vi "Compare.vi"(4 "gB":dbl, 6 "fB":dbl, 9 "gA":dbl, 10 "fA":dbl, 11 "Priority Queue in":refnum<class "NI_Robotics_Priority Queue.lvclass">) -> (2 "priority(A) > priority(B)":bool, 3 "Priority Queue out":refnum<class "NI_Robotics_Priority Queue.lvclass">)   [LabVIEW 2017, in "NI_Robotics_Priority Queue.lvclass"]
uses:
  <vilib>/robotics/Navigation/shared/Priority Queue/NI_Robotics_Priority Queue.lvclass
  <vilib>/robotics/Navigation/shared/Priority Queue/NI_Robotics_Priority Queue.lvclass/NI_Robotics_Priority Queue.ctl
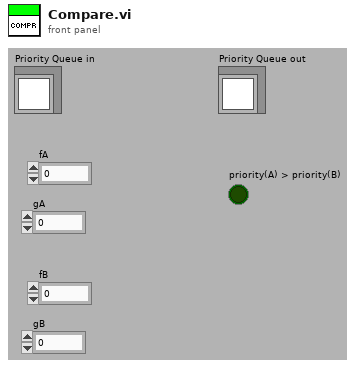
[diagram p1: front panel]
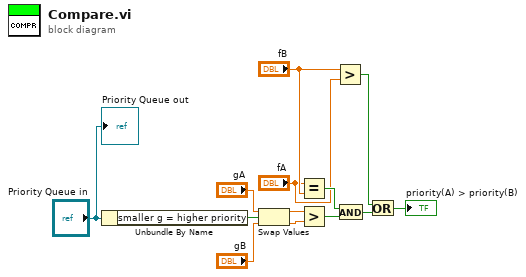
[diagram p0: block diagram]
diagram:
  n1 = Unbundle By Name("Priority Queue in") -> ("smaller g = higher priority"=w13:bool)
  n2 = Swap Values(12:"gA", 13:w13, 14:"gB") -> (1:w5:dbl, 3:w4:dbl)
  n3 = Equal?(x="fA", y="fB") -> (x = y?=w10:bool)
  n4 = Greater?(x=w5, y=w4) -> (0:w2:bool)
  n5 = Greater?(x="fB", y="fA") -> (0:w1:bool)
  n6 = And(x=w10, y=w2) -> (x .and. y?=w11:bool)
  n7 = Or(x=w1, y=w11) -> (x .or. y?=→"priority(A) > priority(B)":bool)
  "Priority Queue out" <- "Priority Queue in"
